vi "PlayfieldStatusCheck.vi"(9 "TetroInfo Input":T1, 11 "Playfield":bool[][](array[boolean])) -> (0 "isGameOver":bool, 1 "TetroInfo Output":T1)   [LabVIEW 2026]
uses:
  02_StateMachine/GameTetrominoInformationTypeDef.ctl
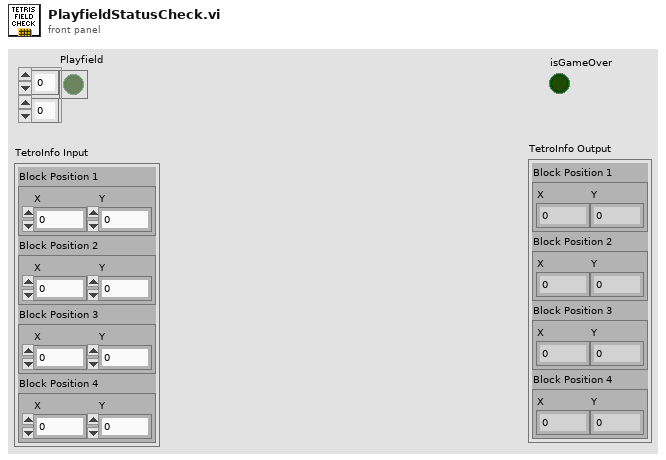
[diagram p1: front panel]
types:
  T1 = typedef "GameTetrominoInformationTypeDef.ctl" = cluster{"Block Position 1":cluster{"X":i32, "Y":i32}, "Block Position 2":cluster{"X":i32, "Y":i32}, "Block Position 3":cluster{"X":i32, "Y":i32}, "Block Position 4":cluster{"X":i32, "Y":i32}}
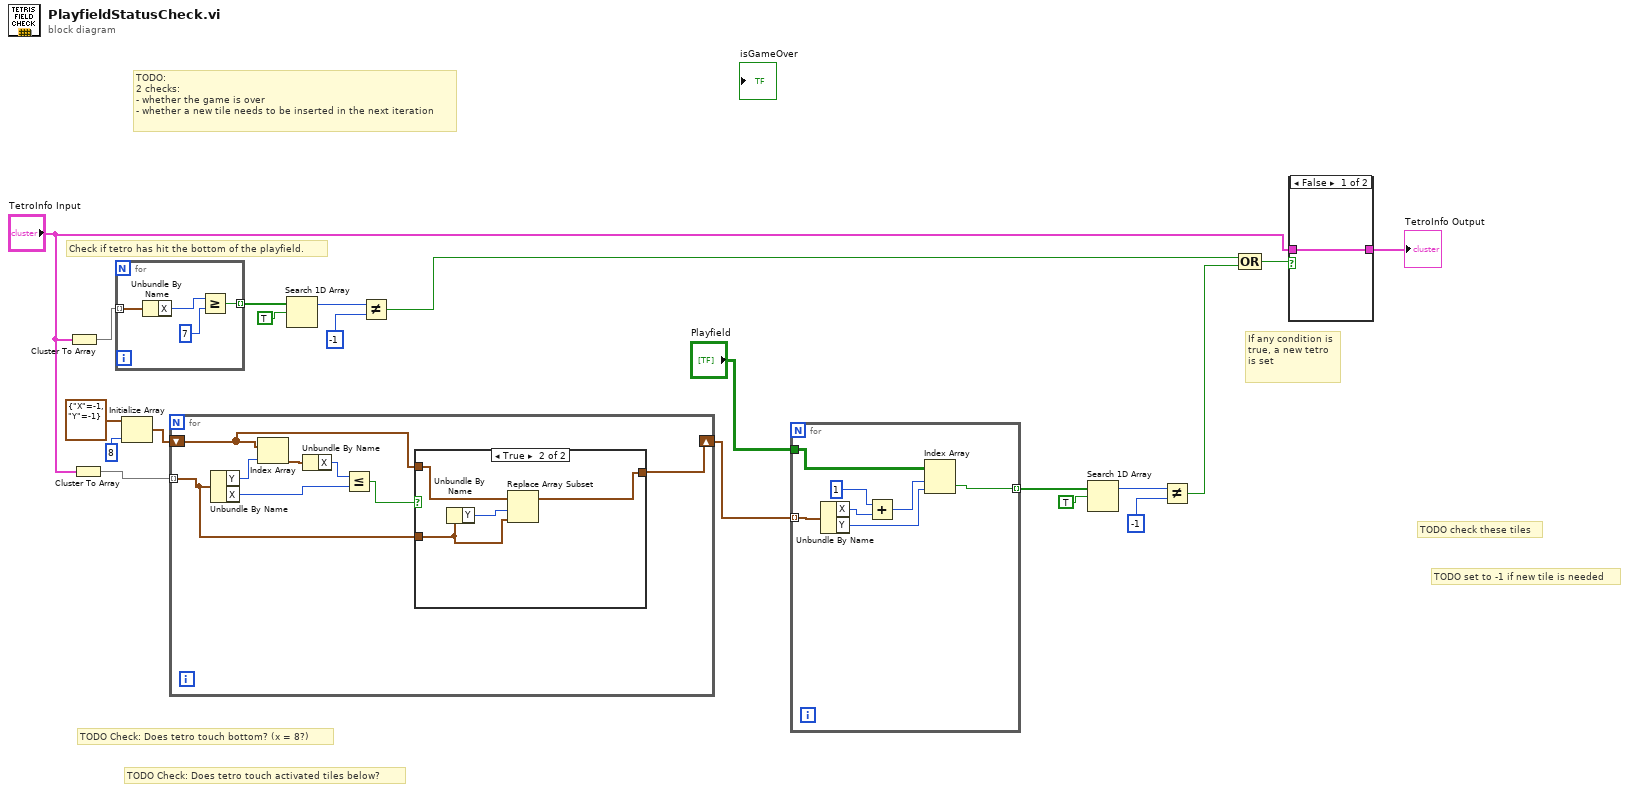
[diagram p0: block diagram]
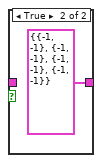
[diagram p3: hidden frame]
diagram:
  # "TODO check these tiles"
  # "Check if tetro has hit the bottom of the playfield."
  # "If any condition is true, a new tetro is set"
  # "TODO Check: Does tetro touch activated tiles below?"
  # "TODO Check: Does tetro touch bottom? (x = 8?)"
  # "TODO:\n2 checks:\n- whether the game is over\n- whether a new tile needs to be inserted in the next iteration"
  # "TODO set to -1 if new tile is needed"
  n1 = Cluster To Array(cluster="TetroInfo Input") -> (array=w18:cluster{"X":i32, "Y":i32}[])
  n2 = Cluster To Array(cluster="TetroInfo Input") -> (array=w11:cluster{"X":i32, "Y":i32}[])
  n3 = for {
    tunnel: w18 -> [w24] mode=indexing
    tunnel: [w23] -> w17 mode=indexing
    n4 = Unbundle By Name(w24) -> ("X"=w22:i32)
    n5 = Greater Or Equal?(x=w22, y=7 ("x")) -> (x >= y?=w23:bool)
  }
  n6 = Initialize Array(cluster{"X":i32, "Y":i32} {"X"=-1, "Y"=-1}, 8 ("dimension size")) -> (w8:cluster{"X":i32, "Y":i32}[])
  n7 = for {
    tunnel: w11 -> [w29] mode=indexing
    shift-right: [w27] -> w7
    shift-left: w8 -> [w28]
    n8 = Unbundle By Name(w29) -> ("Y"=w32:i32, "X"=w31:i32)
    n9 = Index Array(array=w28, index=w32) -> (element=w26:cluster{"X":i32, "Y":i32})
    n10 = Unbundle By Name(w26) -> ("X"=w25:i32)
    n11 = Less Or Equal?(x=w25, y=w31) -> (x <= y?=w30:bool)
    n12 = case shown="True" w30 {
      tunnel: w29 -> [_ w34]
      tunnel: w28 -> [w33 w37]
      tunnel: [w33 w36] -> w27
      frame False {
      }
      frame True {
        n13 = Unbundle By Name(w34) -> ("Y"=w35:i32)
        n14 = Replace Array Subset(array=w37, new element=w34, index=w35) -> (w36:cluster{"X":i32, "Y":i32}[])
      }
    }
  }
  n15 = Search 1D Array(1D array=w17, element=TRUE) -> (index of element=w15:i32)  [unwired: 1 in]
  n16 = Not Equal?(x=w15, y=-1) -> (x != y?=w13:bool)
  n17 = for {
    tunnel: w7 -> [w44] mode=indexing
    tunnel: "Playfield" -> [w41]
    tunnel: [w38] -> w2 mode=indexing
    n18 = Unbundle By Name(w44) -> ("X"=w43:i32, "Y"=w39:i32)
    n19 = Add(x=1, y=w43) -> (x+y=w40:i32)
    n20 = Index Array(array=w41, index (row)=w40, index (col)=w39) -> (element=w38:bool)
  }
  n21 = Search 1D Array(1D array=w2, element=TRUE) -> (index of element=w4:i32)  [unwired: 1 in]
  n22 = Not Equal?(x=w4, y=-1) -> (x != y?=w1:bool)
  n23 = Compound Arithmetic op=OR(w13, w1) -> (w19:bool)
  n24 = case shown="False" w19 {
    tunnel: "TetroInfo Input" -> [w45 _]
    tunnel: [w45 T1 {"Block Position 1"={"X"=-1, "Y"=-1}, "Block Position 2"={"X"=-1, "Y"=-1}, "Block Position 3"={"X"=-1, "Y"=-1}, "Block Position 4"={"X"=-1, "Y"=-1}} ("TetroInfo")] -> w20
    frame False {
    }
    frame True {
    }
  }
  "TetroInfo Output" <- w20
